vi "Angle Changer.vi"(3 "Angle":dbl) -> (0 "dt output":dbl, 1 "Output":dbl)   [LabVIEW 2018]
uses:
  <vilib>/Rock Robotics/WPI/ThirdParty/Sensors/navX/_TypeDefs/FRIC_navX_DeviceNumbersTypeDef.ctl
  <vilib>/addons/control/pid/pid.llb/PID (DBL).vi
  <vilib>/addons/control/pid/NI_PID_pid.lvlib
panel:
  in  "Range":cluster{"MAX":dbl, "MIN":dbl}
  in  "dt":dbl
  in  "PID Gains":cluster{"P":dbl, "I":dbl, "D":dbl}
  # "seconds"
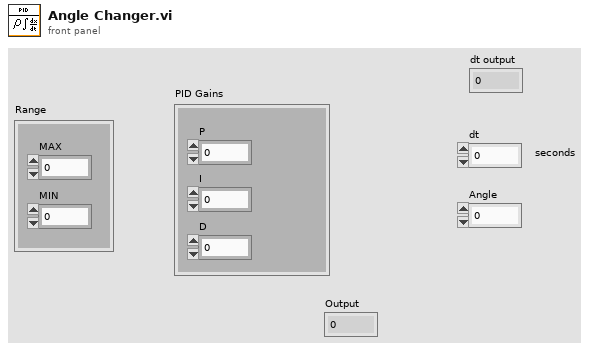
[diagram p1: front panel]
types:
  T1 = typedef "FRIC_navX_DeviceNumbersTypeDef.ctl" = enum16{"Dev0", "Dev1", "Dev2", "Dev3"}
  T2 = cluster{"Yaw":dbl, "Roll":dbl, "Pitch":dbl, "Heading":dbl, "Fused Heading":dbl}
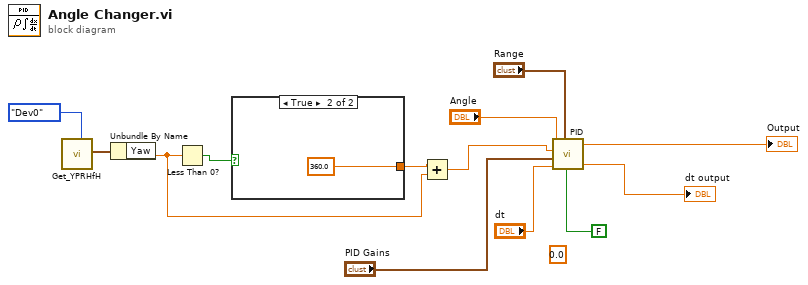
[diagram p0: block diagram]
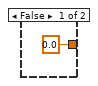
[diagram p2: hidden frame]
diagram:
  (unwired) 0.0
  n1 = call <vilib>:"Get_YPRHfH.vi"("Device Number"=FRIC_navX_DeviceNumbersTypeDef."Dev0") -> ("YRPHfH"=w12:T2)  [unwired: 10 in]
  n2 = Unbundle By Name(w12) -> ("Yaw"=w3:dbl)
  n3 = Less Than 0?(x=w3) -> (x < 0?=w4:bool)
  n4 = case shown="True" w4 {
    tunnel: [0.0 360.0] -> w2
    frame False {
    }
    frame True {
    }
  }
  n5 = Add(x=w2, y=w3) -> (x+y=w1:dbl)
  n6 = call-poly <vilib>:"PID.vi"("reinitialize? (F)"=FALSE, "output range"="Range", "dt (s)"="dt", "PID gains"="PID Gains", "process variable"=w1, "setpoint"="Angle") -> ("dt out (s)"=→"dt output":dbl, "output"=→"Output":dbl)  [unwired: 4 in]
